vi "(TestVI)example_scope_producer consumer architecture.vi"() -> ()   [LabVIEW 2020]
uses:
  Serial/Controls/(Ctrl)Serial_FGV Function.ctl
panel:
  in  "Register":u16[](array[numeric])=[0] format="%.0x"
  in  "정지":bool
  out "Scope_Data":i32[][](graph) caption="Data"
  in  "User Code":u8
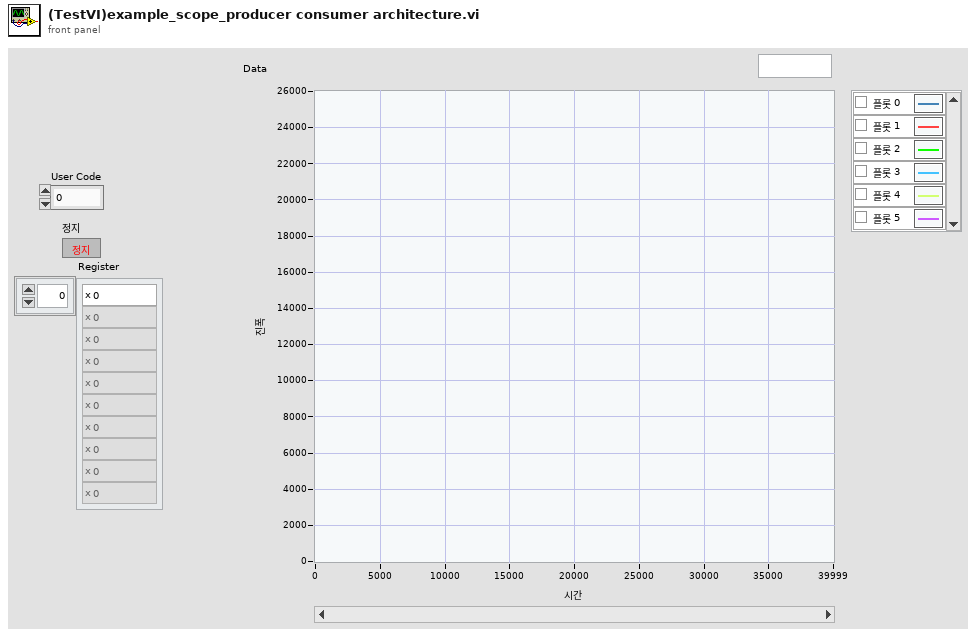
[diagram p1: front panel]
types:
  T1 = typedef "(Ctrl)Serial_FGV Function.ctl" = enum16{"Initialize", "Read", "Read All", "Write", "Flush Buffer", "Get Ref.", "Close"}
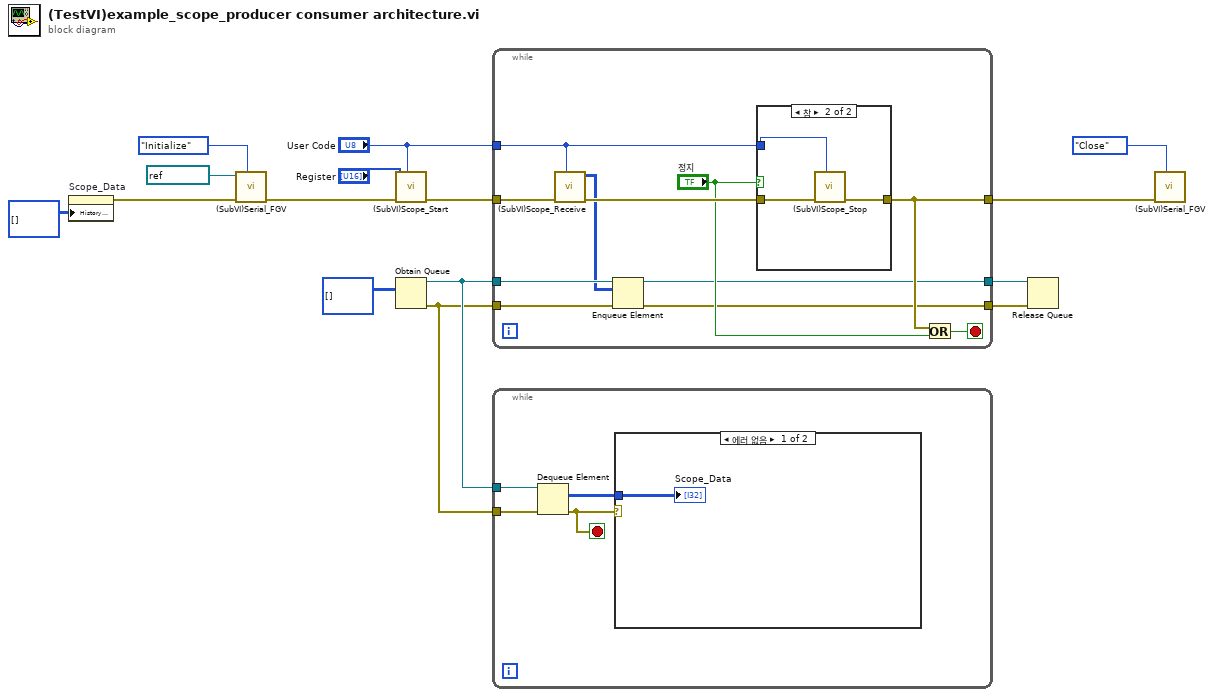
[diagram p0: block diagram]
diagram:
  n1 = property on="Scope_Data" class="WFChart (엄격한)"("History Data"=i32[][] [] ("히스토리 데이터")) -> (error out=w3:errorcluster)  [unwired: 2 in, 1 out]
  n2 = call "(SubVI)Serial_FGV.vi"("Function"=(Ctrl)Serial_FGV_Function."Initialize", "error in (no error)"=w3, "VISA resource name"=refnum<visa-resource-name> "COM3") -> ("error out"=w12:errorcluster)  [unwired: 6 in, 2 out]
  n3 = call "(SubVI)Scope_Start.vi"("Mode"="User Code", "error in (no error)"=w12, "Recording Time"="Register") -> ("error out"=w5:errorcluster)  [unwired: 8 in]
  n4 = Obtain Queue(element data type=i32[][] [] ("Data")) -> (queue out=w7:refnum<queue>, error out=w1:errorcluster)  [unwired: 4 in, 1 out]
  n5 = while {
    tunnel: "User Code" -> [w24]
    tunnel: w7 -> [w20]
    tunnel: w5 -> [w26]
    tunnel: [w21] -> w11
    tunnel: [w18] -> w6
    tunnel: w1 -> [w17]
    tunnel: [w16] -> w4
    stop <- w22 stop-if-true
    n6 = call "(SubVI)Scope_Receive.vi"("User Code"=w24, "error in (no error)"=w26) -> ("error out"=w25:errorcluster, "Data"=w19:i16[][])  [unwired: 7 in, 1 out]
    n7 = Enqueue Element(queue=w20, element=w19, error in (no error)=w17) -> (queue out=w18:refnum<queue>, error out=w16:errorcluster)  [unwired: 1 in, 1 out]
    n8 = case shown="참" "정지" {
      tunnel: w25 -> [w27 w30]
      tunnel: [w27 w29] -> w21
      tunnel: w24 -> [_ w28]
      frame False {
      }
      frame True {
        n9 = call "(SubVI)Scope_Stop.vi"(7:w28, "error in (no error)"=w30) -> ("error out"=w29:errorcluster)  [unwired: 9 in]
      }
    }
    n10 = Or(x=w21, y="정지") -> (x .or. y?=w22:bool)
  }
  n11 = while {
    tunnel: w7 -> [w34]
    tunnel: w1 -> [w33]
    stop <- w32 stop-if-true
    n12 = Dequeue Element(queue=w34, error in (no error)=w33) -> (element=w31:i32[][], error out=w32:errorcluster)  [unwired: 1 in, 2 out]
    n13 = case shown="에러 없음" w32 {
      tunnel: w31 -> [w35 _]
      frame No Error {
        "Scope_Data" <- w35
      }
      frame Error {
      }
    }
  }
  n14 = Release Queue(queue=w6, error in (no error)=w4) -> ()  [unwired: 1 in, 3 out]
  n15 = call "(SubVI)Serial_FGV.vi"("Function"=(Ctrl)Serial_FGV_Function."Close", "error in (no error)"=w11) -> ()  [unwired: 7 in, 3 out]
